vi "Write Response Msg.vi"(10 "Serial.lvlib:Response Msg.lvclass":refnum<class "Response Msg.lvclass">, 11 "Serial in":refnum<class "Serial.lvclass">) -> (3 "Serial out":refnum<class "Serial.lvclass">)   [LabVIEW 2019, in "Serial.lvlib" / "Serial.lvclass"]
uses:
  Serial.lvclass
  Serial Messages/Response Msg/Response Msg.lvclass
  Serial.lvclass/Serial.ctl
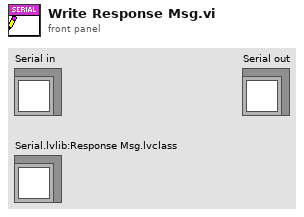
[diagram p1: front panel]
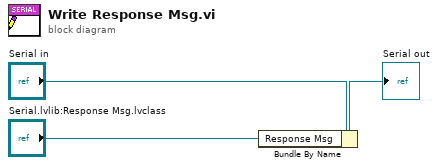
[diagram p0: block diagram]
diagram:
  n1 = Bundle By Name(cluster="Serial in", "Response Msg"="Serial.lvlib:Response Msg.lvclass") -> (→"Serial out":refnum<class "Serial.lvclass">)
